vi "proptest_supportedtargets.vi"() -> ()   [LabVIEW 2013, in "TBM Tests.lvlib"]
uses:
  TBM Tests.lvlib
  root configuration/TBM configuration.lvclass
panel:
  out "error 538305":errorcluster
  out "no support=ok":bool
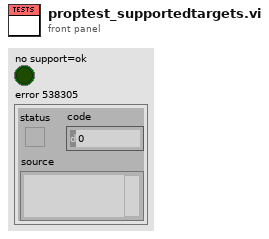
[diagram p1: front panel]
types:
  T1 = typedef "TBM configuration.lvclass/Target Types.ctl" = enum16{"Windows", "Mac", "Linux", "Linux RT ARM", "VxWorks", "Pharlap", "Other", "Linux RT x64"}
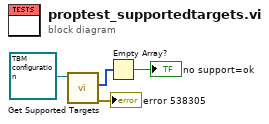
[diagram p0: block diagram]
diagram:
  n1 = call-dynamic "Get Supported Targets.vi"("configuration in"=refnum<class "TBM configuration.lvclass"> refnum ("configuration")) -> ("error out"=→"error 538305":errorcluster, "supported targets"=w2:T1[])  [unwired: 8 in, 1 out]
  n2 = Empty Array?(array=w2) -> (empty?=→"no support=ok":bool)
